vi "Teleop.vi"(10 "Match Info":T1={"Autonomous Elapsed Seconds"=0.0, "TeleOp Elapsed Seconds"=0.0, "Disabled Elapsed Seconds"=0.0, "Visited Autonomous"=FALSE, "Visited TeleOp"=FALSE, "Visited Disabled"=FALSE, "Autonomous Settings"={"Autonomous Style"=enum."Independent", "VI Refnum"=refnum}}, 11 "Call Context":T2) -> ()   [LabVIEW 2014]
doc: "This VI is called for each TeleOp packet received from the DS where the robot is not disabled. It is often used to read from the joysticks and update I/O or to update setpoints for timed control loops. It should complete and return within 20 milliseconds or it may miss DS packets."
uses:
  <vilib>/Rock Robotics/WPI/DriverStation/WPI_DriverStationDerivedRobotMode.ctl
  <vilib>/Rock Robotics/WPI/DriverStation/WPI_DriverStationMatch Info.ctl
  DriverButtons.ctl
  OpAxis.ctl
  OpButtons.ctl
  DriverAxis.ctl
  Global Ref.vi
  <vilib>/Rock Robotics/Network Tables/SD Write Boolean.vi
  Robot Values.vi
  DriveGlobal.vi
  Robot Fail.vi
  <vilib>/Rock Robotics/Network Tables/SD Write Numeric Array.vi
  <vilib>/Rock Robotics/Network Tables/SD Read Boolean.vi
  <vilib>/Rock Robotics/Network Tables/SD Write Boolean Array.vi
  <vilib>/Rock Robotics/Network Tables/SD Read Number.vi
panel:
  out "Sample Slider 0":dbl(slide) scale=0.0..5.0
  out "Sample Boolean 1":bool
  out "Sample Boolean 0":bool
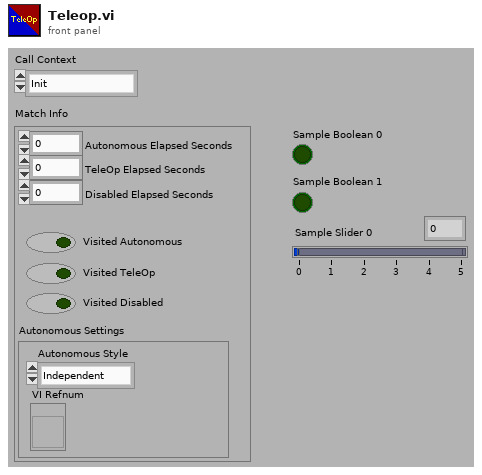
[diagram p1: front panel]
types:
  T1 = typedef "WPI_DriverStationMatch Info.ctl" = cluster{"Autonomous Elapsed Seconds":dbl, "TeleOp Elapsed Seconds":dbl, "Disabled Elapsed Seconds":dbl, "Visited Autonomous":bool, "Visited TeleOp":bool, "Visited Disabled":bool, "Autonomous Settings":cluster{"Autonomous Style":enum16{"Iterative", "Independent"}, "VI Refnum":refnum<vi>}}
  T2 = typedef "WPI_DriverStationDerivedRobotMode.ctl" = enum16{"Init", "Execute", "Stop"}
  T3 = typedef "OpButtons.ctl" = cluster{"Lift Pos 1":bool, "Lift Pos 2":bool, "Lift Pos 3":bool, "Lift Pos 4":bool, "Left Bumper":bool, "Right Bumper":bool, "Boolean 7":bool, "Boolean 8":bool, "Boolean9":bool, "Lift override":bool, "Boolean 11":bool, "Boolean 12":bool}
  T4 = typedef "OpAxis.ctl" = cluster{"Left X":dbl, "Left Y":dbl, "Right X":dbl, "Right Y":dbl, "D-Pad X":dbl, "D-Pad Y":dbl}
  T5 = typedef "DriverButtons.ctl" = cluster{"ToteAutokeep":bool, "ToteAutoSpit":bool, "Boolean 3":bool, "TrackTote":bool, "ToteLeftspit":bool, "ToteRigthspit":bool, "ToteLeftPull":bool, "Control power":bool, "Drive mode":bool, "Boolean 10":bool, "Boolean 11":bool, "ToteRightPull":bool}
  T6 = typedef "DriverAxis.ctl" = cluster{"Left X":dbl, "Left Y":dbl, "Right X":dbl, "Right Y":dbl, "D-Pad X":dbl, "D-Pad Y":dbl}
  T7 = cluster{"Left X":dbl, "Left Y":dbl, "Trigger L":dbl, "Trigger R":dbl, "Right X":dbl, "Right Y":dbl}
  T8 = typedef "WPI_RobotDriveDevRef.ctl" = cluster{"DevStatus":errorcluster, "Motors[]":T9[], "Square Inputs":bool, "Max Output":dbl}
  T9 = typedef "WPI_MotorControlDeviceRef.ctl" = cluster{"DeviceStatus":errorcluster, "Type":T10, "PWM":cluster{"Controller":T11, "PWM Channel":T12, "DeadBand":T13}, "CAN":cluster{"Device Number":u8, "Control Mode":T14, "Semaphore":T15, "Max Vout":dbl, "TalonSRX Control Mode":T16}, "Invert":bool, "TransformRef":T17, "InvTransformRef":T17}
  T10 = typedef "WPI_MotorControlType.ctl" = enum16{"PWM", "CAN", "CANTalonSRX"}
  T11 = typedef "FPGA_TypedefDigitalModule.ctl" = enum16{"Controller 1"}
  T12 = typedef "FPGA_DIOPWMChannel.ctl" = enum8{"PWM 0", "PWM 1", "PWM 2", "PWM 3", "PWM 4", "PWM 5", "PWM 6", "PWM 7", "PWM 8", "PWM 9", "PWM MXP 0", "PWM MXP 1", "PWM MXP 2", "PWM MXP 3", "PWM MXP 4", "PWM MXP 5", "PWM MXP 6", "PWM MXP 7", "PWM MXP 8", "PWM MXP 9", "Invalid"}
  T13 = typedef "WPI_PWMDeadband.ctl" = cluster{"Name":string, "maxPositivePwm":i32, "minPositivePwm":i32, "centerPwm":i32, "maxNegativePwm":i32, "minNegativePwm":i32, "angularRange":u16}
  T14 = typedef "WPI_CANJaguar_ControlMode.ctl" = enum8{"Percent VBus", "Current", "Speed", "Position", "Voltage"}
  T15 = typedef "Semaphore RefNum" = refnum<k1>
  T16 = typedef "WPI_CANTalonSRX_APIControlMode.ctl" = enum8{"Percent VBus", "Speed", "Position", "Slave", "Unchanged / Invalid"}
  T17 = typedef "WPI_PWMTransform_ConPane.ctl" = refnum<vi>
  T18 = typedef "WPI_JoystickDevRef.ctl" = cluster{"Device":T19}
  T19 = typedef "WPI_JoystickDeviceEnum.ctl" = enum16{"USB 0", "USB 1", "USB 2", "USB 3", "USB 4", "USB 5"}
  T20 = typedef "Global Ref typedef.ctl" = cluster{"Drive":cluster{"RobotDriveDevRef":T8}, "Joysticks":cluster{"JoyDriveRef":T18, "JoyOpRef":T18, "JoySabatourRef":T18}, "Lift":cluster{"LiftMotorRefLeft":T9, "LiftMotorRefRight":T9}, "Lift Limits":cluster{"Bottom Left":T21, "Bottom Right":T21}, "Accel":cluster{"AccelerometerDevRef":T23}, "Lift Encoder":cluster{"AIDeviceRefRight":T32, "AIDeviceRefLeft":T32}, "Lights":cluster{"Swag Light Ref cluster":cluster{"PWMDeviceRef1":T33, "PWMDeviceRef2":T33, "PWMDeviceRef3":T33, "PWMDeviceRef4":T33, "PWMDeviceRef5":T33, "PWMDeviceRef6":T33, "PWMDeviceRef7":T33, "PWMDeviceRef8":T33}}, "Camera":cluster{"GrayScaleImage":T34, "ColorImage":T34, "CameraDevRef":T35}, "Drive Encoders":cluster{"AIDeviceRef Left":T32, "AIDeviceRef Right":T32}, "Gyro":cluster{"GyroDevRef":T36}, "Relay":cluster{"RelayDevRef":T37, "RelayDevRef 2":T37}, "Gripper Arm Motors":cluster{"Gripper Arm Left":T9, "Gripper Arm Right":T9}, "Gripper Arm Limit":cluster{"Gripper Limit Left":T21, "Gripper Limit Right":T21}}
  T21 = typedef "WPI_DigitalInputDevRef.ctl" = cluster{"DevStatus":errorcluster, "DIO Channel":T22, "Controller":T11}
  T22 = typedef "FPGA_DIOChannel.ctl" = enum8{"DIO 0", "DIO 1", "DIO 2", "DIO 3", "DIO 4", "DIO 5", "DIO 6", "DIO 7", "DIO 8", "DIO 9", "DIO MXP 0", "DIO MXP 1", "DIO MXP 2", "DIO MXP 3", "DIO MXP 4", "DIO MXP 5", "DIO MXP 6", "DIO MXP 7", "DIO MXP 8", "DIO MXP 9", "DIO MXP 10", "DIO MXP 11", "DIO MXP 12", "DIO MXP 13", "DIO MXP 14", "DIO MXP 15", "Invalid"}
  T23 = typedef "WPI_AccelerometerDevRef.ctl" = cluster{"DevStatus":errorcluster, "Controller":T24, "Scaling":T25, "Analog Channels":T26, "I2C Bus":T28, "SPI Bus":T29, "Accel Range":T30, "ADXL345 Axes":T31, "Handle":i32, "Device Address":u8, "Accel Type":enum16{"Analog", "ADXL345 I2C", "ADXL345 SPI", "Internal"}}
  T24 = typedef "FPGA_TypedefAnalogModule.ctl" = enum16{"Controller 1"}
  T25 = typedef "WPI_AccelerometerScaling.ctl" = cluster{"Gain (VoltsPerG)":dbl, "Center Voltage":dbl}
  T26 = typedef "WPI_AccelerometerAnalogChannels.ctl" = cluster{"X-Axis":T27, "Y-Axis":T27, "Z-Axis":T27}
  T27 = typedef "FPGA_AIChannel.ctl" = enum8{"AI 0", "AI 1", "AI 2", "AI 3", "AI MXP 0", "AI MXP 1", "AI MXP 2", "AI MXP 3", "Invalid"}
  T28 = typedef "i2c_bus.ctl" = enum16{"I2C On-Board", "I2C MXP", "Invalid"}
  T29 = typedef "spi_bus.ctl" = enum16{"SPI On-Board, CS0", "SPI On-Board, CS1", "SPI On-Board, CS2", "SPI On-Board, CS3", "SPI MXP", "Invalid"}
  T30 = typedef "ADXL345 Range.ctl" = u8
  T31 = typedef "WPI_AccelerometerADXL345 Axes.ctl" = cluster{"X-Axis":bool, "Y-Axis":bool, "Z-Axis":bool}
  T32 = typedef "WPI_AnalogChannelDevRef.ctl" = cluster{"DevStatus":errorcluster, "Controller":T24, "Analog Channel":T27}
  T33 = typedef "WPI_PWMDeviceRef.ctl" = cluster{"DeviceStatus":errorcluster, "Controller":T11, "PWM Channel":T12}
  T34 = typedef "IMAQ Image.ctl" = refnum<image>
  T35 = typedef "WPI_CameraDevRef.ctl" = cluster{"Camera Address":string, "CameraStatus":errorcluster}
  T36 = typedef "WPI_GyroDevRef.ctl" = cluster{"DevStatus":errorcluster, "Analog Module":T24, "Analog Channel":T27, "Offset":dbl, "Gain (VoltsPerDegree/Second)":dbl}
  T37 = typedef "WPI_RelayDevRef.ctl" = cluster{"DevStatus":errorcluster, "Relay Channel":T38, "Controller":T11, "Relay Direction":T39}
  T38 = typedef "FPGA_DIORelayChannel.ctl" = enum8{"Relay 0", "Relay 1", "Relay 2", "Relay 3", "Invalid"}
  T39 = typedef "WPI_RelayDirection.ctl" = enum16{"Both directions", "Forward only", "Reverse only"}
  T40 = cluster{"DriveMode":enum16{"Tank", "Arcade"}, "Is Logitech":bool}
  T41 = cluster{"Tracking Tote?":bool, "ToteRightSpeed":dbl, "ToteLeftSpeed":dbl, "Drive Encoder reset":bool, "Right Wheel \n(Cm)":dbl, "Left Wheel \n(Cm)":dbl}
  T42 = cluster{"Lift Position":i32, "Lift Speed Override":dbl, "OverrideTele?":bool, "OverrideDash":bool}
  T43 = cluster{"RightMotorSpeed":dbl, "LeftMotorSpeed":dbl}
  T44 = cluster{"Not stright - Right":bool, "Not stright - Left":bool, "Lift position change":bool, "Lift out of sync":bool, "Joystick sensitivity Less":bool, "Stuck in Tank":bool, "Joystick Sensistiviy More":bool}
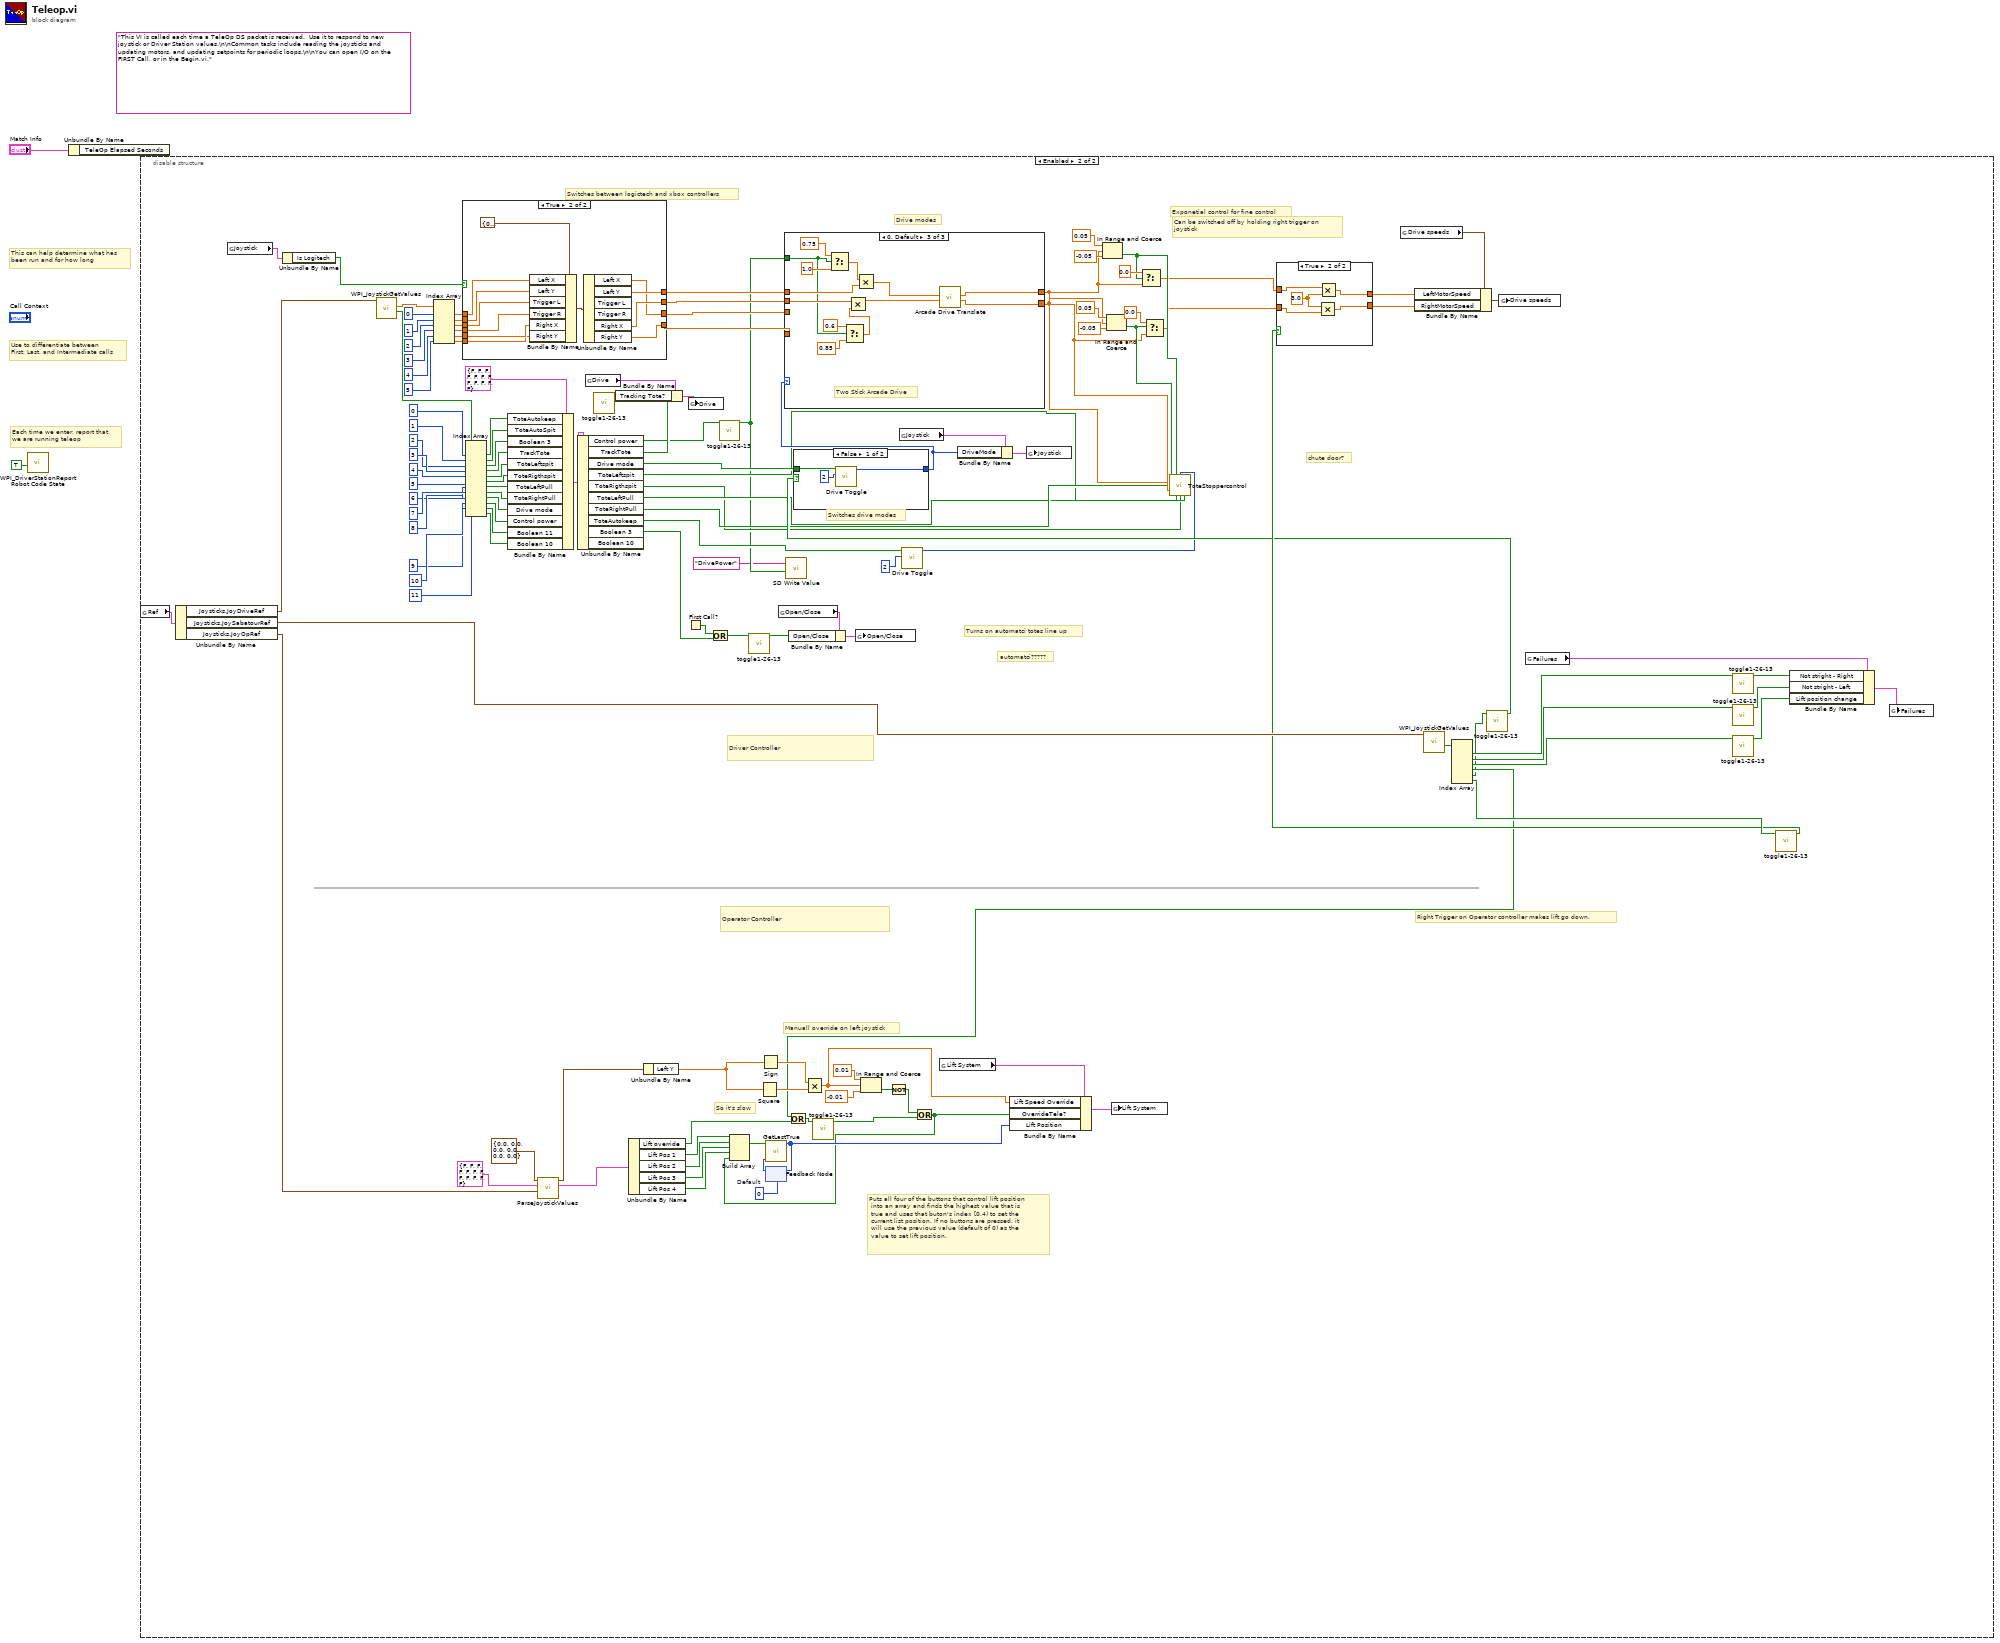
[diagram p0: block diagram]
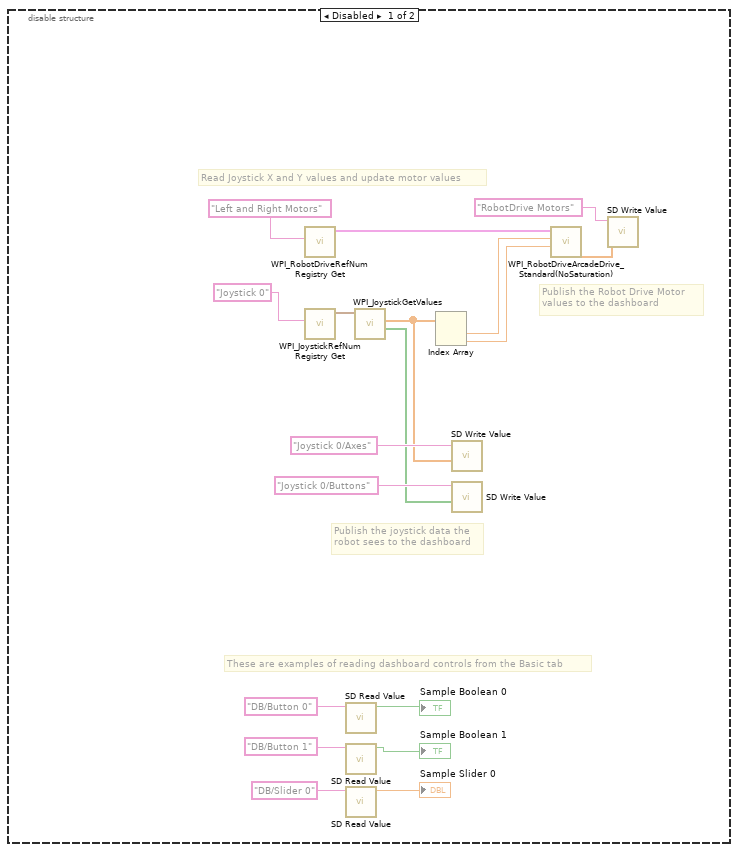
[diagram p2: hidden frame]
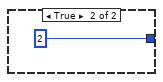
[diagram p3: hidden frame]
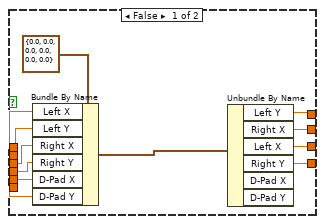
[diagram p5: hidden frame]
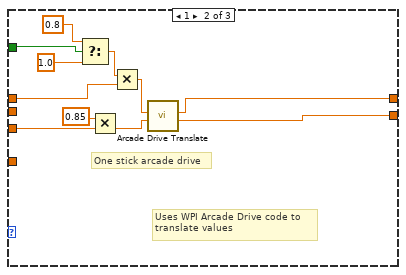
[diagram p7: hidden frame]
diagram:
  (unwired) "This VI is called each time a TeleOp DS packet is received.  Use it to respond to new joystick or Driver Station values.\n\nCommon tasks include reading the joysticks and updating motors, and updating setpoints for periodic loops.\n\nYou can open I/O on the FIRST Call, or in the Begin.vi."
  # "Each time we enter, report that\nwe are running teleop"
  # "Use to differentiate between\nFirst, Last, and Intermediate calls"
  # "This can help determine what has\nbeen run and for how long"
  n1 = call <vilib>:"WPI_DriverStationReport Robot Code State.vi"("TeleOp"=TRUE ("Autonomous")) -> ()  [unwired: 10 in, 1 out]
  n2 = Unbundle By Name("Match Info") -> ()  [unwired: 1 out]
  n3 = disable-structure shown="Enabled" {
    frame Disabled {
      # "These are examples of reading dashboard controls from the Basic tab"
      # "Publish the Robot Drive Motor\nvalues to the dashboard"
      # "Publish the joystick data the\nrobot sees to the dashboard"
      # "Read Joystick X and Y values and update motor values"
      n4 = call <vilib>:"WPI_RobotDriveRefNum Registry Get.vi"("refnum name"="Left and Right Motors") -> ("RobotDriveDevRef"=w19:T8)  [unwired: 1 in, 9 out]
      n5 = call <vilib>:"WPI_JoystickRefNum Registry Get.vi"("refnum name"="Joystick 0") -> ("JoystickDevRef"=w16:T18)  [unwired: 1 in, 9 out]
      n6 = call-poly <vilib>:"SD Read Value.vi"("Name"="DB/Button 0" ("refnum name")) -> ("Boolean"=→"Sample Boolean 0":bool)  [unwired: 8 in, 2 out]
      n7 = call-poly <vilib>:"SD Read Value.vi"("Name"="DB/Button 1" ("refnum name")) -> ("Boolean"=→"Sample Boolean 1":bool)  [unwired: 8 in, 2 out]
      n8 = call-poly <vilib>:"SD Read Value.vi"("Name"="DB/Slider 0" ("refnum name")) -> ("Numeric"=→"Sample Slider 0":dbl)  [unwired: 8 in, 2 out]
      n9 = call <vilib>:"WPI_JoystickGetValues.vi"("JoystickDevRef"=w16) -> ("Buttons"=w3:bool[], "Axes"=w5:dbl[])  [unwired: 6 in, 3 out]
      n10 = Index Array(array=w5) -> (element #1=w18:dbl, element #2=w8:dbl)  [unwired: 2 in]
      n11 = call-poly <vilib>:"SD Write Value.vi"("Numeric Array"=w5, "Name"="Joystick 0/Axes") -> ()  [unwired: 8 in, 2 out]
      n12 = call-poly <vilib>:"SD Write Value.vi"("Boolean Array"=w3, "Name"="Joystick 0/Buttons") -> ()  [unwired: 8 in, 2 out]
      n13 = call <vilib>:"WPI_RobotDriveArcadeDrive_Standard(NoSaturation).vi"("Y axis value"=w8, "X axis value"=w18, "RobotDriveDevRef"=w19) -> ("Motor Values"=w7:dbl[])  [unwired: 1 in, 7 out]
      n14 = call-poly <vilib>:"SD Write Value.vi"("Numeric Array"=w7, "Name"="RobotDrive Motors") -> ()  [unwired: 8 in, 2 out]
    }
    frame Enabled {
      w90 = 0  # Default
      # "chute door?"
      # "automatci?????"
      # "Right Trigger on Operator controller makes lift go down."
      # "Manuall override on left joystick"
      # "Switches drive modes"
      # "Turns on automatci totes line up"
      # "Can be switched off by holding right trigger on \njoystick"
      # "Exponetial control for fine control"
      # "Drive modes"
      # "Switches between logictech and xbox controllers"
      # "So it's slow"
      # "Puts all four of the buttons that control lift position\n into an array and finds the highest value that is \n true and uses that buton's index [0,4) to set the\n current list position. If no buttons are pressed, it\n will use the previous value (default of 0) as the\n value to set lift position."
      # "Driver Controller"
      # "Operator Controller"
      n15 = global read "Global Ref.vi" "Ref"() -> (w150:T20)
      n16 = Unbundle By Name(w150) -> ("Joysticks.JoyDriveRef"=w94:T18, "Joysticks.JoySabatourRef"=w61:T18, "Joysticks.JoyOpRef"=w146:T18)
      n17 = global read "Robot Values.vi" "Joystick"() -> (w80:T40)
      n18 = Unbundle By Name(w80) -> ("Is Logitech"=w79:bool)
      n19 = call <vilib>:"WPI_JoystickGetValues.vi"("JoystickDevRef"=w94) -> ("Buttons"=w134:bool[], "Axes"=w108:dbl[])  [unwired: 6 in, 3 out]
      n20 = Index Array(array=w108, index #1=0 ("index"), index #2=1 ("index"), index #3=2 ("index"), index #4=3 ("index"), index #5=4 ("index"), index #6=5 ("index")) -> (element #1=w102:dbl, element #2=w103:dbl, element #3=w104:dbl, element #4=w105:dbl, element #5=w106:dbl, element #6=w107:dbl)
      n21 = case shown="True" w79 {
        tunnel: w107 -> [w173 w179]
        tunnel: w106 -> [w172 w180]
        tunnel: w105 -> [w171 w181]
        tunnel: w104 -> [w170 w182]
        tunnel: w103 -> [w169 w183]
        tunnel: w102 -> [w168 w184]
        tunnel: [w165 w177] -> w84
        tunnel: [w164 w176] -> w83
        tunnel: [w163 w174] -> w82
        tunnel: [w162 w175] -> w81
        frame False {
          n22 = Bundle By Name(cluster=T6 {"Left X"=0.0, "Left Y"=0.0, "Right X"=0.0, "Right Y"=0.0, "D-Pad X"=0.0, "D-Pad Y"=0.0} ("input cluster"), "Left X"=w168, "Left Y"=w169, "Right X"=w170, "Right Y"=w171, "D-Pad X"=w172, "D-Pad Y"=w173) -> (w167:T6)
          n23 = Unbundle By Name(w167) -> ("Left Y"=w165:dbl, "Right X"=w164:dbl, "Left X"=w162:dbl, "Right Y"=w163:dbl)  [unwired: 2 out]
        }
        frame True {
          n24 = Bundle By Name(cluster=T7 {"Left X"=0.0, "Left Y"=0.0, "Trigger L"=0.0, "Trigger R"=0.0, "Right X"=0.0, "Right Y"=0.0} ("Xbox Axis"), "Left X"=w184, "Left Y"=w183, "Trigger L"=w182, "Trigger R"=w181, "Right X"=w180, "Right Y"=w179) -> (w178:T7)
          n25 = Unbundle By Name(w178) -> ("Left X"=w175:dbl, "Left Y"=w177:dbl, "Right X"=w176:dbl, "Right Y"=w174:dbl)  [unwired: 2 out]
        }
      }
      n26 = Index Array(array=w134, index #1=0 ("index"), index #2=1 ("index"), index #3=2 ("index"), index #4=3 ("index"), index #5=4 ("index"), index #6=5 ("index"), index #7=6 ("index"), index #8=7 ("index"), index #9=8 ("index"), index #10=9 ("index"), index #11=10 ("index"), index #12=11 ("index")) -> (element #1=w122:bool, element #2=w123:bool, element #3=w124:bool, element #4=w125:bool, element #5=w126:bool, element #6=w127:bool, element #7=w128:bool, element #8=w129:bool, element #9=w130:bool, element #10=w131:bool, element #11=w132:bool, element #12=w133:bool)
      n27 = Bundle By Name(cluster=T5 {"ToteAutokeep"=FALSE, "ToteAutoSpit"=FALSE, "Boolean 3"=FALSE, "TrackTote"=FALSE, "ToteLeftspit"=FALSE, "ToteRigthspit"=FALSE, "ToteLeftPull"=FALSE, "Control power"=FALSE, "Drive mode"=FALSE, "Boolean 10"=FALSE, "Boolean 11"=FALSE, "ToteRightPull"=FALSE} ("Cluster"), "ToteAutokeep"=w122, "ToteAutoSpit"=w123, "Boolean 3"=w124, "TrackTote"=w125, "ToteLeftspit"=w126, "ToteRigthspit"=w127, "ToteLeftPull"=w128, "ToteRightPull"=w129, "Drive mode"=w130, "Control power"=w131, "Boolean 11"=w132, "Boolean 10"=w133) -> (w96:T5)
      n28 = call "ParseJoystickValues.vi"("JoyRef"=w146, "Button Names"=T3 {"Lift Pos 1"=FALSE, "Lift Pos 2"=FALSE, "Lift Pos 3"=FALSE, "Lift Pos 4"=FALSE, "Left Bumper"=FALSE, "Right Bumper"=FALSE, "Boolean 7"=FALSE, "Boolean 8"=FALSE, "Boolean9"=FALSE, "Lift override"=FALSE, "Boolean 11"=FALSE, "Boolean 12"=FALSE} ("input cluster"), "Axis Names"=T4 {"Left X"=0.0, "Left Y"=0.0, "Right X"=0.0, "Right Y"=0.0, "D-Pad X"=0.0, "D-Pad Y"=0.0} ("input cluster")) -> ("Named Button Values"=w137:T3, "Named Axis Values"=w138:T4)  [unwired: 7 in]
      n29 = Unbundle By Name(w96) -> ("Control power"=w36:bool, "TrackTote"=w88:bool, "Drive mode"=w93:bool, "ToteLeftspit"=w32:bool, "ToteRigthspit"=w33:bool, "ToteLeftPull"=w34:bool, "ToteRightPull"=w35:bool, "ToteAutokeep"=w27:bool, "Boolean 3"=w26:bool)  [unwired: 1 out]
      n30 = global read "Robot Values.vi" "Drive"() -> (w87:T41)
      n31 = call "toggle1-26-13.vi"("input"=w88) -> ("output"=w85:bool)  [unwired: 10 in]
      n32 = Bundle By Name(cluster=w87, "Tracking Tote?"=w85) -> (w86:T41)
      n33 = Unbundle By Name(w137) -> ("Lift override"=w69:bool, "Lift Pos 1"=w145:bool, "Lift Pos 2"=w144:bool, "Lift Pos 3"=w143:bool, "Lift Pos 4"=w142:bool)
      n34 = Unbundle By Name(w138) -> ("Left Y"=w78:dbl)
      n35 = First Call?() -> (First Call?: T/F=w23:bool)
      n36 = global write "Robot Values.vi" "Drive"(w86) -> ()
      n37 = Or(x=w23, y=w26) -> (x .or. y?=w24:bool)
      n38 = call "toggle1-26-13.vi"("input"=w36) -> ("output"=w22:bool)  [unwired: 10 in]
      n39 = call "toggle1-26-13.vi"("input"=w24) -> ("output"=w25:bool)  [unwired: 10 in]
      n40 = Square(x=w78) -> (x^2=w89:dbl)
      n41 = Sign(1:w78) -> (0:w77:dbl)
      n42 = feedback #1(w90) -> (w91:i32)
      n43 = global read "Robot Values.vi" "Open/Close"() -> (w29:cluster{"Open/Close":bool})
      n44 = call-poly <vilib>:"SD Write Value.vi"("Boolean"=w22, "Name"="DrivePower") -> ()  [unwired: 8 in, 2 out]
      n45 = Bundle By Name(cluster=w29, "Open/Close"=w25) -> (w28:cluster{"Open/Close":bool})
      n46 = Multiply(x=w77, y=w89) -> (x*y=w74:dbl)
      n47 = global write "Robot Values.vi" "Open/Close"(w28) -> ()
      n48 = In Range and Coerce(upper limit=0.01, x=w74, lower limit=-0.01) -> (In Range?=w73:bool)  [unwired: 1 out]
      n49 = Not(x=w73) -> (.not. x?=w72:bool)
      n50 = global read "Robot Values.vi" "Joystick"() -> (w149:T40)
      n51 = call "Drive Toggle.vi"("Limit"=2, "Button"=w27) -> ("Output"=w31:i32)  [unwired: 9 in]
      n52 = global read "Robot Values.vi" "Lift System"() -> (w140:T42)
      n53 = global read "DriveGlobal.vi" "Drive speeds"() -> (w70:T43)
      n54 = call <vilib>:"WPI_JoystickGetValues.vi"("JoystickDevRef"=w61) -> ("Buttons"=w60:bool[])  [unwired: 6 in, 4 out]
      n55 = Index Array(array=w60) -> (element #1=w57:bool, element #2=w56:bool, element #3=w55:bool, element #4=w46:bool, element #5=w45:bool, element #6=w49:bool)  [unwired: 6 in]
      n56 = Or(x=w46, y=w69) -> (x .or. y?=w47:bool)
      n57 = call "toggle1-26-13.vi"("input"=w47) -> ("output"=w68:bool)  [unwired: 10 in]
      n58 = Or(x=w72, y=w68) -> (x .or. y?=w39:bool)
      n59 = Build Array(w145, w144, w143, w142, w39) -> (w92:bool[])
      n60 = call "GetLastTrue.vi"("Default value"=w91, "Input"=w92) -> ("Last True"=w139:i32)  [unwired: 9 in]
      n61 = feedback-in #1(w139) -> ()
      n62 = Bundle By Name(cluster=w140, "Lift Speed Override"=w74, "OverrideTele?"=w39, "Lift Position"=w139) -> (w141:T42)
      n63 = global write "Robot Values.vi" "Lift System"(w141) -> ()
      n64 = call "toggle1-26-13.vi"("input"=w45) -> ("output"=w44:bool)  [unwired: 10 in]
      n65 = case shown="False" w44 {
        tunnel: [w152 2 ("Output")] -> w147
        tunnel: w93 -> [w151 _]
        frame False {
          n66 = call "Drive Toggle.vi"("Limit"=2, "Button"=w151) -> ("Output"=w152:i32)  [unwired: 9 in]
        }
        frame True {
        }
      }
      n67 = case shown="0, Default" w147 {
        tunnel: w84 -> [w187 w193 w207]
        tunnel: w83 -> [_ _ w209]
        tunnel: w82 -> [w186 _ _]
        tunnel: w81 -> [_ w196 _]
        tunnel: [w187 w198 w211] -> w40
        tunnel: [w186 w197 w210] -> w41
        tunnel: w22 -> [_ w188 w202]
        frame 2 {
          # "This is Tank Drive"
          # "Gets joystick values and saves\nthem to the Robot Values typedef"
        }
        frame 1 {
          # "One stick arcade drive"
          # "Uses WPI Arcade Drive code to\ntranslate values"
          n68 = Select(t=0.8, s=w188, f=1.0 ("x")) -> (s? t:f=w189:dbl)
          n69 = Multiply(x=0.85, y=w196) -> (x*y=w195:dbl)
          n70 = Multiply(x=w189, y=w193) -> (x*y=w192:dbl)
          n71 = call "Arcade Drive Translate.vi"("xAxis"=w195, "yAxis"=w192) -> ("outputX"=w197:dbl, "outputY"=w198:dbl)  [unwired: 7 in]
        }
        frame 0, Default {
          # "Two Stick Arcade Drive"
          n72 = Select(t=0.75, s=w202, f=1.0 ("x")) -> (s? t:f=w204:dbl)
          n73 = Select(t=0.6 ("y"), s=w202, f=0.85) -> (s? t:f=w201:dbl)
          n74 = Multiply(x=w209, y=w201) -> (x*y=w208:dbl)
          n75 = Multiply(x=w204, y=w207) -> (x*y=w206:dbl)
          n76 = call "Arcade Drive Translate.vi"("xAxis"=w208, "yAxis"=w206) -> ("outputX"=w210:dbl, "outputY"=w211:dbl)  [unwired: 7 in]
        }
      }
      n77 = Bundle By Name(cluster=w149, "DriveMode"=w147) -> (w148:T40)
      n78 = global write "Robot Values.vi" "Joystick"(w148) -> ()
      n79 = In Range and Coerce(upper limit=0.05, x=w40, lower limit=-0.05) -> (In Range?=w43:bool)  [unwired: 1 out]
      n80 = In Range and Coerce(upper limit=0.05, x=w41, lower limit=-0.05) -> (In Range?=w42:bool)  [unwired: 1 out]
      n81 = Select(t=0.0, s=w43, f=w40) -> (s? t:f=w38:dbl)
      n82 = Select(t=0.0, s=w42, f=w41) -> (s? t:f=w37:dbl)
      n83 = call "ToteStoppercontrol.vi"("Right moving"=w42, "Left moving?"=w43, "Last True"=w31, "outputY"=w40, "ToteRightPull"=w35, "outputX"=w41, "ToteLeftspit"=w32, "ToteRigthspit"=w33, "ToteLeftPull"=w34) -> ()  [unwired: 7 in]
      n84 = global read "Robot Fail.vi" "Failures"() -> (w58:T44)
      n85 = call "toggle1-26-13.vi"("input"=w57) -> ("output"=w54:bool)  [unwired: 10 in]
      n86 = call "toggle1-26-13.vi"("input"=w56) -> ("output"=w53:bool)  [unwired: 10 in]
      n87 = call "toggle1-26-13.vi"("input"=w55) -> ("output"=w52:bool)  [unwired: 10 in]
      n88 = call "toggle1-26-13.vi"("input"=w49) -> ("output"=w48:bool)  [unwired: 10 in]
      n89 = case shown="True" w48 {
        tunnel: w38 -> [w156 w160]
        tunnel: w37 -> [w155 w161]
        tunnel: [w156 w159] -> w51
        tunnel: [w155 w158] -> w50
        frame False {
        }
        frame True {
          w157 = 3.0
          n90 = Multiply(x=w157, y=w161) -> (x*y=w158:dbl)
          n91 = Multiply(x=w160, y=w157) -> (x*y=w159:dbl)
        }
      }
      n92 = Bundle By Name(cluster=w70, "LeftMotorSpeed"=w51, "RightMotorSpeed"=w50) -> (w71:T43)
      n93 = global write "DriveGlobal.vi" "Drive speeds"(w71) -> ()
      n94 = Bundle By Name(cluster=w58, "Not stright - Right"=w54, "Not stright - Left"=w53, "Lift position change"=w52) -> (w59:T44)
      n95 = global write "Robot Fail.vi" "Failures"(w59) -> ()
    }
  }
